vi "Set Menu for View Selection.vi"(8 "error in":errorcluster, 10 "String":string, 11 "Menu in":refnum<k9>) -> (2 "Value":T1)   [LabVIEW 2019, in "CML UI.lvlib"]
uses:
  CML UI.lvlib
  UI Tab Select.ctl
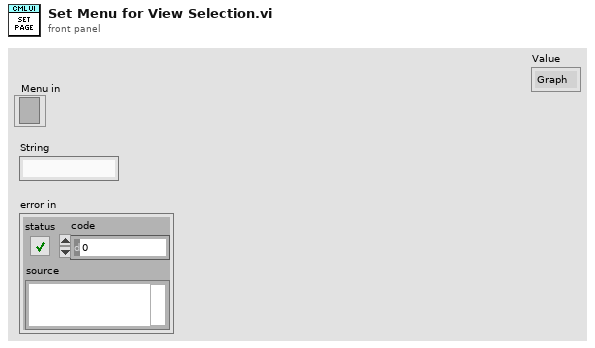
[diagram p1: front panel]
types:
  T1 = typedef "CML UI.lvlib/UI Tab Select.ctl" = enum32{"Graph", "Impedance", "More Options", "Single Graph", "CNV Demo", "Eyes O/C Demo"}
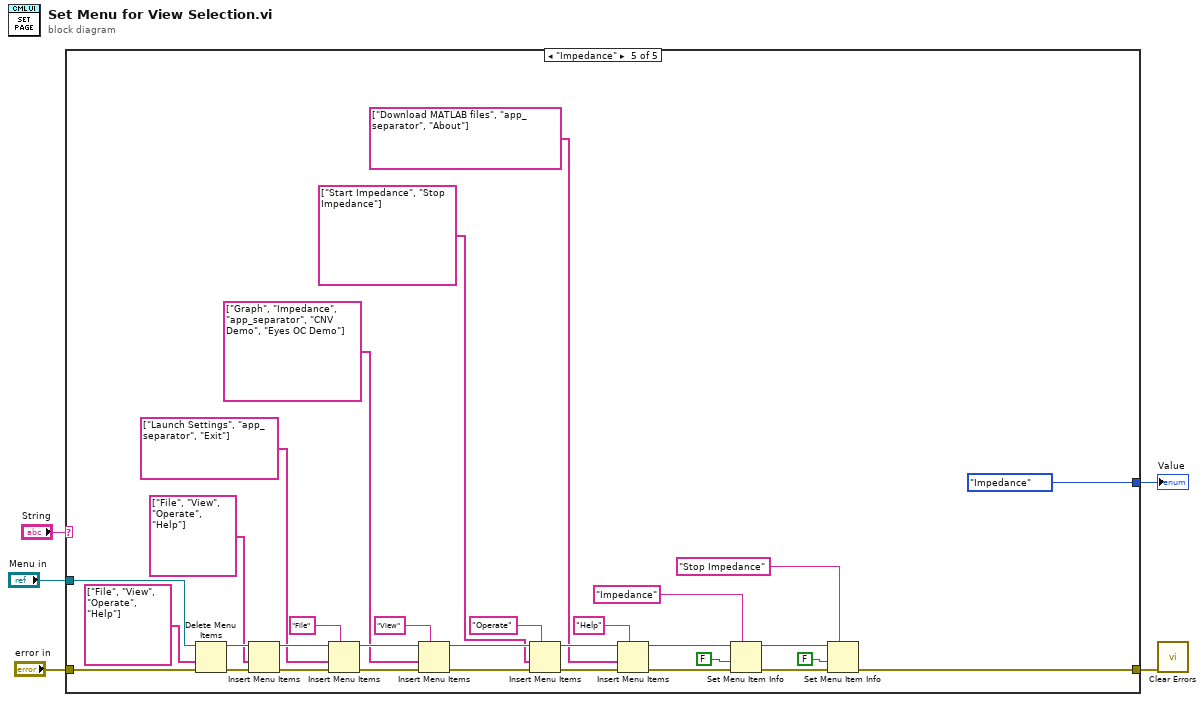
[diagram p0: block diagram]
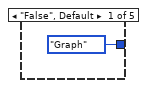
[diagram p2: hidden frame]
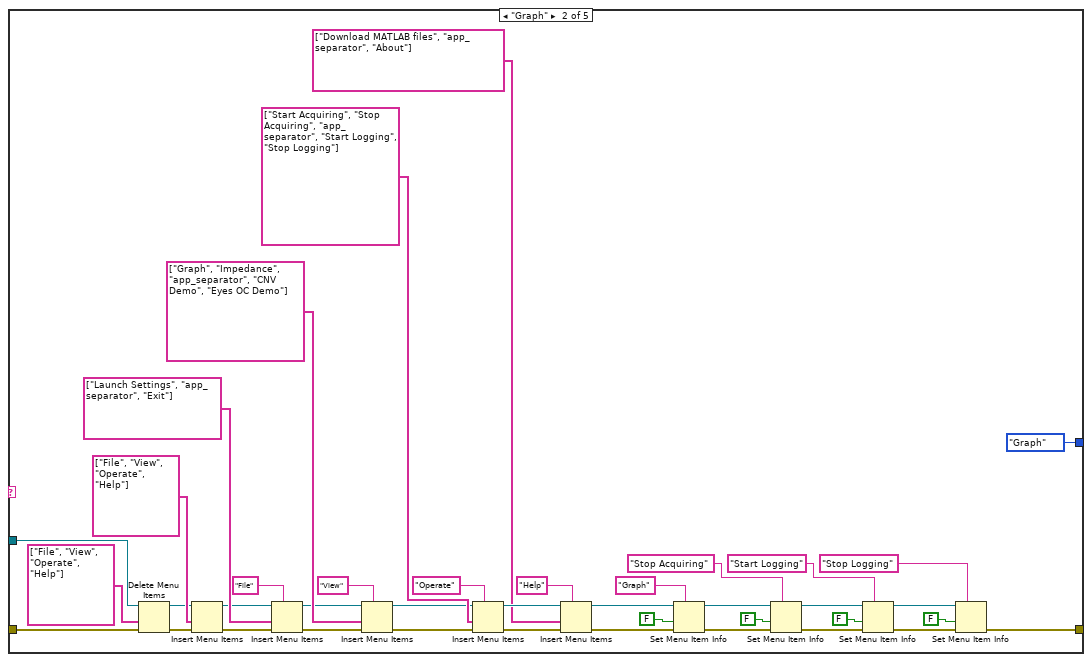
[diagram p3: hidden frame]
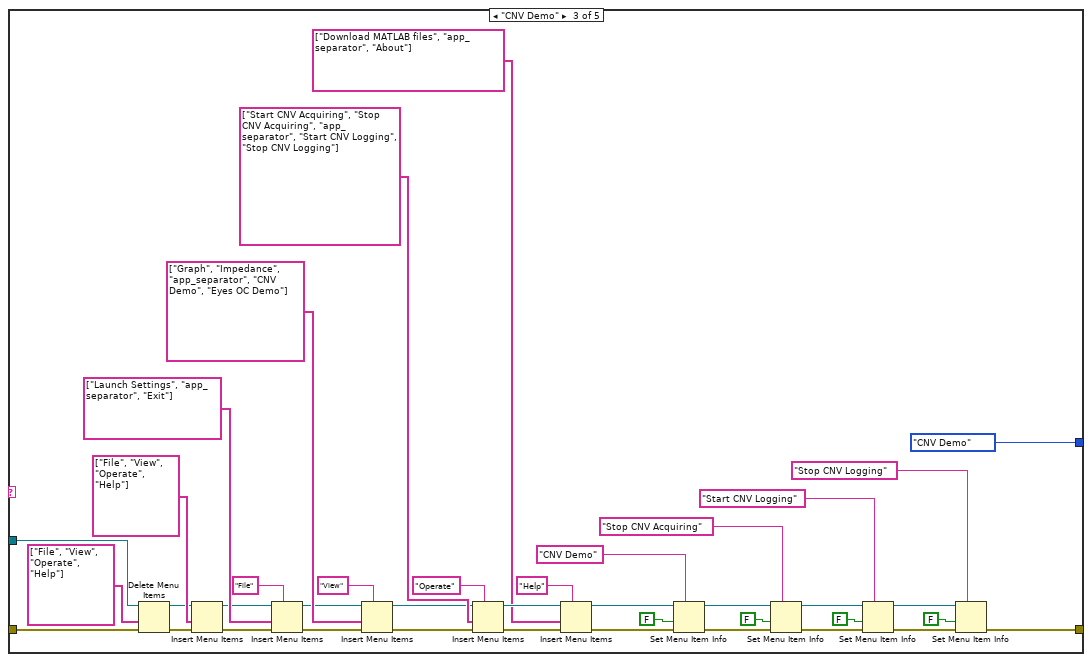
[diagram p4: hidden frame]
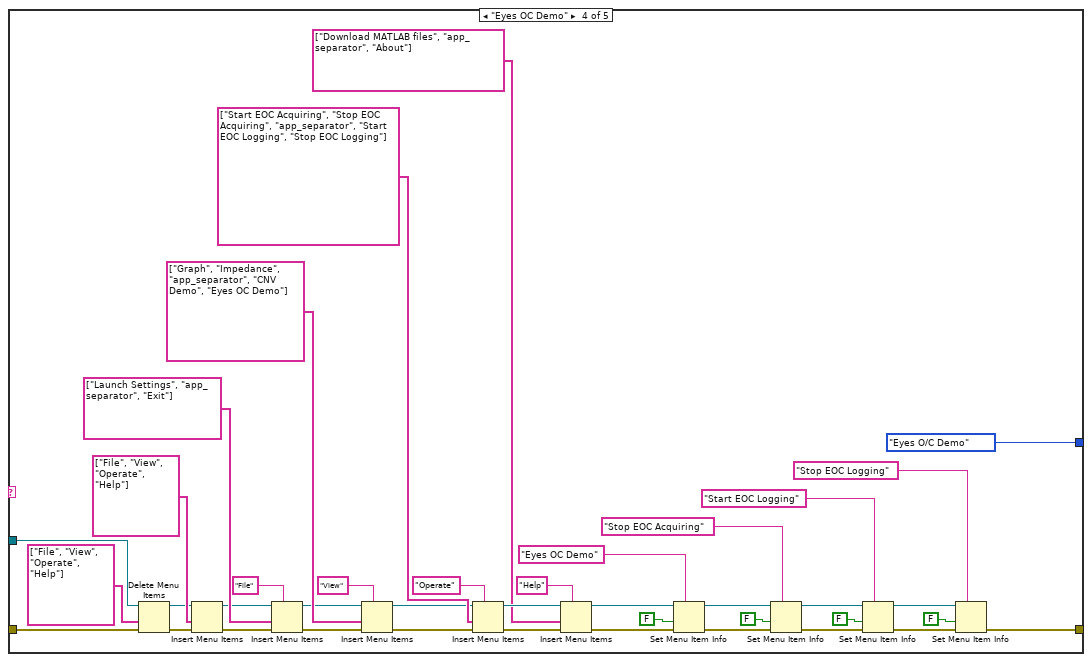
[diagram p5: hidden frame]
diagram:
  n1 = case shown="\"Impedance\"" "String" {
    tunnel: [UI_Tab_Select."Graph" ("Value") UI_Tab_Select."Graph" ("Value") UI_Tab_Select."CNV Demo" ("Value") UI_Tab_Select."Eyes O/C Demo" ("Value") UI_Tab_Select."Impedance" ("Value")] -> w1
    tunnel: "Menu in" -> [_ w9 w50 w90 w129]
    tunnel: "error in" -> [_ w10 w49 w89 w130]
    tunnel: [_ w23 w51 w103 w156] -> w5
    frame "False", Default {
    }
    frame "Graph" {
      n2 = Delete Menu Items(6:w10, 7:string[] ["File", "View", "Operate", "Help"] ("L10n_item tags 1"), 9:w9) -> (0:w21:errorcluster, 3:w22:refnum<k9>)  [unwired: 1 in]
      n3 = Insert Menu Items(6:w21, 7:string[] ["File", "View", "Operate", "Help"] ("L10n_item tags 1"), 9:w22) -> (0:w35:errorcluster, 3:w33:refnum<k9>)  [unwired: 3 in, 1 out]
      n4 = Insert Menu Items(5:"File" ("L10n_menu tag"), 6:w35, 7:string[] ["Launch Settings", "app_separator", "Exit"] ("L10n_item tags 2"), 9:w33) -> (0:w40:errorcluster, 3:w39:refnum<k9>)  [unwired: 2 in, 1 out]
      n5 = Insert Menu Items(5:"View" ("L10n_menu tag"), 6:w40, 7:string[] ["Graph", "Impedance", "app_separator", "CNV Demo", "Eyes OC Demo"] ("L10n_item tags 2"), 9:w39) -> (0:w44:errorcluster, 3:w43:refnum<k9>)  [unwired: 2 in, 1 out]
      n6 = Insert Menu Items(5:"Operate" ("L10n_menu tag"), 6:w44, 7:string[] ["Start Acquiring", "Stop Acquiring", "app_separator", "Start Logging", "Stop Logging"] ("L10n_item tags 2"), 9:w43) -> (0:w30:errorcluster, 3:w31:refnum<k9>)  [unwired: 2 in, 1 out]
      n7 = Insert Menu Items(5:"Help" ("L10n_menu tag"), 6:w30, 7:string[] ["Download MATLAB files", "app_separator", "About"] ("L10n_item tags 2"), 9:w31) -> (0:w27:errorcluster, 3:w29:refnum<k9>)  [unwired: 2 in, 1 out]
      n8 = Set Menu Item Info(7:"Graph" ("item tag"), 8:w27, 9:FALSE ("enabled"), 11:w29) -> (0:w15:errorcluster, 3:w16:refnum<k9>)  [unwired: 3 in]
      n9 = Set Menu Item Info(7:"Stop Acquiring" ("item tag"), 8:w15, 9:FALSE ("enabled"), 11:w16) -> (0:w13:errorcluster, 3:w14:refnum<k9>)  [unwired: 3 in]
      n10 = Set Menu Item Info(7:"Start Logging" ("item tag"), 8:w13, 9:FALSE ("enabled"), 11:w14) -> (0:w11:errorcluster, 3:w12:refnum<k9>)  [unwired: 3 in]
      n11 = Set Menu Item Info(7:"Stop Logging" ("item tag"), 8:w11, 9:FALSE ("enabled"), 11:w12) -> (0:w23:errorcluster)  [unwired: 3 in, 1 out]
    }
    frame "CNV Demo" {
      n12 = Delete Menu Items(6:w49, 7:string[] ["File", "View", "Operate", "Help"] ("L10n_item tags 1"), 9:w50) -> (0:w60:errorcluster, 3:w61:refnum<k9>)  [unwired: 1 in]
      n13 = Insert Menu Items(6:w60, 7:string[] ["File", "View", "Operate", "Help"] ("L10n_item tags 1"), 9:w61) -> (0:w75:errorcluster, 3:w73:refnum<k9>)  [unwired: 3 in, 1 out]
      n14 = Insert Menu Items(5:"File" ("L10n_menu tag"), 6:w75, 7:string[] ["Launch Settings", "app_separator", "Exit"] ("L10n_item tags 2"), 9:w73) -> (0:w80:errorcluster, 3:w79:refnum<k9>)  [unwired: 2 in, 1 out]
      n15 = Insert Menu Items(5:"View" ("L10n_menu tag"), 6:w80, 7:string[] ["Graph", "Impedance", "app_separator", "CNV Demo", "Eyes OC Demo"] ("L10n_item tags 2"), 9:w79) -> (0:w84:errorcluster, 3:w83:refnum<k9>)  [unwired: 2 in, 1 out]
      n16 = Insert Menu Items(5:"Operate" ("L10n_menu tag"), 6:w84, 7:string[] ["Start CNV Acquiring", "Stop CNV Acquiring", "app_separator", "Start CNV Logging", "Stop CNV Logging"] ("L10n_item tags 2"), 9:w83) -> (0:w70:errorcluster, 3:w71:refnum<k9>)  [unwired: 2 in, 1 out]
      n17 = Insert Menu Items(5:"Help" ("L10n_menu tag"), 6:w70, 7:string[] ["Download MATLAB files", "app_separator", "About"] ("L10n_item tags 2"), 9:w71) -> (0:w67:errorcluster, 3:w69:refnum<k9>)  [unwired: 2 in, 1 out]
      n18 = Set Menu Item Info(7:"CNV Demo" ("item tag"), 8:w67, 9:FALSE ("enabled"), 11:w69) -> (0:w62:errorcluster, 3:w63:refnum<k9>)  [unwired: 3 in]
      n19 = Set Menu Item Info(7:"Stop CNV Acquiring" ("item tag"), 8:w62, 9:FALSE ("enabled"), 11:w63) -> (0:w52:errorcluster, 3:w53:refnum<k9>)  [unwired: 3 in]
      n20 = Set Menu Item Info(7:"Start CNV Logging" ("item tag"), 8:w52, 9:FALSE ("enabled"), 11:w53) -> (0:w59:errorcluster, 3:w58:refnum<k9>)  [unwired: 3 in]
      n21 = Set Menu Item Info(7:"Stop CNV Logging" ("item tag"), 8:w59, 9:FALSE ("enabled"), 11:w58) -> (0:w51:errorcluster)  [unwired: 3 in, 1 out]
    }
    frame "Eyes OC Demo" {
      n22 = Delete Menu Items(6:w89, 7:string[] ["File", "View", "Operate", "Help"] ("L10n_item tags 1"), 9:w90) -> (0:w101:errorcluster, 3:w102:refnum<k9>)  [unwired: 1 in]
      n23 = Insert Menu Items(6:w101, 7:string[] ["File", "View", "Operate", "Help"] ("L10n_item tags 1"), 9:w102) -> (0:w115:errorcluster, 3:w113:refnum<k9>)  [unwired: 3 in, 1 out]
      n24 = Insert Menu Items(5:"File" ("L10n_menu tag"), 6:w115, 7:string[] ["Launch Settings", "app_separator", "Exit"] ("L10n_item tags 2"), 9:w113) -> (0:w120:errorcluster, 3:w119:refnum<k9>)  [unwired: 2 in, 1 out]
      n25 = Insert Menu Items(5:"View" ("L10n_menu tag"), 6:w120, 7:string[] ["Graph", "Impedance", "app_separator", "CNV Demo", "Eyes OC Demo"] ("L10n_item tags 2"), 9:w119) -> (0:w124:errorcluster, 3:w123:refnum<k9>)  [unwired: 2 in, 1 out]
      n26 = Insert Menu Items(5:"Operate" ("L10n_menu tag"), 6:w124, 7:string[] ["Start EOC Acquiring", "Stop EOC Acquiring", "app_separator", "Start EOC Logging", "Stop EOC Logging"] ("L10n_item tags 2"), 9:w123) -> (0:w110:errorcluster, 3:w111:refnum<k9>)  [unwired: 2 in, 1 out]
      n27 = Insert Menu Items(5:"Help" ("L10n_menu tag"), 6:w110, 7:string[] ["Download MATLAB files", "app_separator", "About"] ("L10n_item tags 2"), 9:w111) -> (0:w107:errorcluster, 3:w109:refnum<k9>)  [unwired: 2 in, 1 out]
      n28 = Set Menu Item Info(7:"Eyes OC Demo" ("item tag"), 8:w107, 9:FALSE ("enabled"), 11:w109) -> (0:w95:errorcluster, 3:w96:refnum<k9>)  [unwired: 3 in]
      n29 = Set Menu Item Info(7:"Stop EOC Acquiring" ("item tag"), 8:w95, 9:FALSE ("enabled"), 11:w96) -> (0:w93:errorcluster, 3:w94:refnum<k9>)  [unwired: 3 in]
      n30 = Set Menu Item Info(7:"Start EOC Logging" ("item tag"), 8:w93, 9:FALSE ("enabled"), 11:w94) -> (0:w91:errorcluster, 3:w92:refnum<k9>)  [unwired: 3 in]
      n31 = Set Menu Item Info(7:"Stop EOC Logging" ("item tag"), 8:w91, 9:FALSE ("enabled"), 11:w92) -> (0:w103:errorcluster)  [unwired: 3 in, 1 out]
    }
    frame "Impedance" {
      n32 = Delete Menu Items(6:w130, 7:string[] ["File", "View", "Operate", "Help"] ("L10n_item tags 1"), 9:w129) -> (0:w158:errorcluster, 3:w157:refnum<k9>)  [unwired: 1 in]
      n33 = Insert Menu Items(6:w158, 7:string[] ["File", "View", "Operate", "Help"] ("L10n_item tags 1"), 9:w157) -> (0:w142:errorcluster, 3:w144:refnum<k9>)  [unwired: 3 in, 1 out]
      n34 = Insert Menu Items(5:"File" ("L10n_menu tag"), 6:w142, 7:string[] ["Launch Settings", "app_separator", "Exit"] ("L10n_item tags 2"), 9:w144) -> (0:w137:errorcluster, 3:w138:refnum<k9>)  [unwired: 2 in, 1 out]
      n35 = Insert Menu Items(5:"View" ("L10n_menu tag"), 6:w137, 7:string[] ["Graph", "Impedance", "app_separator", "CNV Demo", "Eyes OC Demo"] ("L10n_item tags 2"), 9:w138) -> (0:w133:errorcluster, 3:w134:refnum<k9>)  [unwired: 2 in, 1 out]
      n36 = Insert Menu Items(5:"Operate" ("L10n_menu tag"), 6:w133, 7:string[] ["Start Impedance", "Stop Impedance"] ("L10n_item tags 2"), 9:w134) -> (0:w147:errorcluster, 3:w146:refnum<k9>)  [unwired: 2 in, 1 out]
      n37 = Insert Menu Items(5:"Help" ("L10n_menu tag"), 6:w147, 7:string[] ["Download MATLAB files", "app_separator", "About"] ("L10n_item tags 2"), 9:w146) -> (0:w150:errorcluster, 3:w148:refnum<k9>)  [unwired: 2 in, 1 out]
      n38 = Set Menu Item Info(7:"Impedance" ("item tag"), 8:w150, 9:FALSE ("enabled"), 11:w148) -> (0:w155:errorcluster, 3:w154:refnum<k9>)  [unwired: 3 in]
      n39 = Set Menu Item Info(7:"Stop Impedance" ("item tag"), 8:w155, 9:FALSE ("enabled"), 11:w154) -> (0:w156:errorcluster)  [unwired: 3 in, 1 out]
    }
  }
  "Value" <- w1
  n40 = call <vilib>:"Clear Errors.vi"("error in (no error)"=w5) -> ()  [unwired: 5 in, 2 out]
